vi "Get Pi Data.vi"() -> ()   [LabVIEW 2020]
panel:
  out "standard error":string
  out "standard output":string="Active Internet connections (w/o servers)\nProto Recv-Q Send-Q Local Address           Foreign Address         State       \ntcp        0      0 localhost:39876         localhost:41539         ESTABLISHED \ntcp        0    232 192.168.1.102:3079      192.168.1.101:62664     ESTABLISHED \ntcp        0      0 localhost:41539         localhost:39876         ESTABLISHED \nActive UNIX domain sockets (w/o servers)\nProto RefCnt Flags       Type       State         I-Node Path\nunix  2      [ ]         DGRAM                     19720 /run/user/1000/systemd/notify\nunix  4      [ ]         DGRAM                     17418 /var/run/wpa_supplicant/wlan0\nunix  2      [ ]         DGRAM                     17427 /var/run/wpa_supplicant/p2p-dev-wlan0\nunix  2      [ ]         DGRAM                     15198 /tmp/.vncserver-license/0.504\nunix  3      [ ]         DGRAM                      5458 /run/systemd/notify\nunix  2      [ ]         DGRAM                     19551 /run/user/0/systemd/notify\nunix  8      [ ]         DGRAM                      5481 /run/systemd/journal/socket\nunix  20     [ ]         DGRAM                      5493 /run/systemd/journal/dev-log\nunix  2      [ ]         DGRAM                      5517 /run/systemd/journal/syslog\nunix  2      [ ]         DGRAM                     23574 /tmp/dhcpcd-pi/libdhcpcd-wpa-888.0\nunix  2      [ ]         DGRAM                     23575 /tmp/dhcpcd-pi/libdhcpcd-wpa-888.1\nunix  3      [ ]         STREAM     CONNECTED      20302 \nunix  3      [ ]         STREAM     CONNECTED      18013 \nunix  3      [ ]         STREAM     CONNECTED      17093 \nunix  3      [ ]         STREAM     CONNECTED      13957 \nunix  3      [ ]         STREAM     CONNECTED      21078 @/tmp/.X11-unix/X0\nunix  3      [ ]         STREAM     CONNECTED      22652 \nunix  3      [ ]         STREAM     CONNECTED      21440 /run/user/1000/bus\nunix  3      [ ]         STREAM     CONNECTED      20321 @/tmp/.X11-unix/X0\nunix  3      [ ]         STREAM     CONNECTED      19605 /var/run/dbus/system_bus_socket\nunix  3      [ ]         STREAM     CONNECTED      17472 \nunix  2      [ ]         DGRAM                     17271 \nunix  3      [ ]         STREAM     CONNECTED      20299 \nunix  3      [ ]         STREAM     CONNECTED      17782 /run/systemd/journal/stdout\nunix  3      [ ]         STREAM     CONNECTED      14033 \nunix  3      [ ]         STREAM     CONNECTED      17473 /var/run/dbus/system_bus_socket\nunix  3      [ ]         STREAM     CONNECTED      18014 \nunix  3      [ ]         STREAM     CONNECTED      13772 \nunix  3      [ ]         STREAM     CONNECTED      21437 /run/user/1000/bus\nunix  2      [ ]         DGRAM                     17486 \nunix  3      [ ]         STREAM     CONNECTED      20350 /var/run/dbus/system_bus_socket\nunix  2      [ ]         DGRAM                     18729 \nunix  3      [ ]         STREAM     CONNECTED      18114 \nunix  2      [ ]         DGRAM                     17761 \nunix  3      [ ]         STREAM     CONNECTED      13705 \nunix  3      [ ]         STREAM     CONNECTED      18188 /run/systemd/journal/stdout\nunix  2      [ ]         DGRAM                     18697 \nunix  3      [ ]         STREAM     CONNECTED      17270 \nunix  2      [ ]         DGRAM                     13792 \nunix  3      [ ]         STREAM     CONNECTED      21410 \nunix  3      [ ]         STREAM     CONNECTED      18397 /run/user/1000/bus\nunix  3      [ ]         STREAM     CONNECTED      20344 /var/run/dbus/system_bus_socket\nunix  3      [ ]         STREAM     CONNECTED      21127 \nunix  3      [ ]         STREAM     CONNECTED      17009 \nunix  3      [ ]         STREAM     CONNECTED      22631 \nunix  3      [ ]         STREAM     CONNECTED      20264 \nunix  3      [ ]         STREAM     CONNECTED      19600 @/tmp/.X11-unix/X0\nunix  3      [ ]         STREAM     CONNECTED      16668 \nunix  3      [ ]         STREAM     CONNECTED      18410 /run/user/1000/bus\nunix  3      [ ]         STREAM     CONNECTED      18689 \nunix  3      [ ]         STREAM     CONNECTED      18696 \nunix  3      [ ]         STREAM     CONNECTED      17276 \nunix  3      [ ]         STREAM     CONNECTED      17010 /run/systemd/journal/stdout\nunix  3      [ ]         STREAM     CONNECTED      14034 /run/systemd/journal/stdout\nunix  3      [ ]         STREAM     CONNECTED      21326 /run/user/1000/bus\nunix  3      [ ]         STREAM     CONNECTED      22653 \nunix  3      [ ]         STREAM     CONNECTED      22630 \nunix  3      [ ]         STREAM     CONNECTED      16636 \nunix  3      [ ]         STREAM     CONNECTED      14907 \nunix  3      [ ]         STREAM     CONNECTED      14912 /var/run/dbus/system_bus_socket\nunix  3      [ ]         STREAM     CONNECTED      17277 /var/run/dbus/system_bus_socket\nunix  2      [ ]         DGRAM                     16633 \nunix  3      [ ]         STREAM     CONNECTED      18395 /run/systemd/journal/stdout\nunix  3      [ ]         STREAM     CONNECTED      15137 \nunix  3      [ ]         STREAM     CONNECTED      20314 \nunix  3      [ ]         STREAM     CONNECTED      14906 \nunix  3      [ ]         STREAM     CONNECTED      14911 /var/run/dbus/system_bus_socket\nunix  3      [ ]         STREAM     CONNECTED      17094 /run/systemd/journal/stdout\nunix  3      [ ]         STREAM     CONNECTED      14142 \nunix  3      [ ]         STREAM     CONNECTED      21596 /run/user/1000/bus\nunix  3      [ ]         STREAM     CONNECTED      18501 \nunix  2      [ ]         DGRAM                     14137 \nunix  3      [ ]         STREAM     CONNECTED      21604 @/dbus-vfs-daemon/socket-T8U37b0E\nunix  3      [ ]         STREAM     CONNECTED      18128 \nunix  3      [ ]         STREAM     CONNECTED      17437 /run/systemd/journal/stdout\nunix  3      [ ]         STREAM     CONNECTED      21304 /run/user/1000/bus\nunix  3      [ ]         STREAM     CONNECTED      16635 \nunix  3      [ ]         STREAM     CONNECTED      14909 /var/run/dbus/system_bus_socket\nunix  3      [ ]         STREAM     CONNECTED      18910 \nunix  3      [ ]         STREAM     CONNECTED      13774 /run/systemd/journal/stdout\nunix  3      [ ]         STREAM     CONNECTED      18899 \nunix  3      [ ]         STREAM     CONNECTED      17450 /var/run/dbus/system_bus_socket\nunix  2      [ ]         DGRAM                     16602 \nunix  3      [ ]         STREAM     CONNECTED      20311 \nunix  3      [ ]         STREAM     CONNECTED      18909 \nunix  3      [ ]         STREAM     CONNECTED      14118 /run/systemd/journal/stdout\nunix  3      [ ]         STREAM     CONNECTED      19260 /run/user/1000/bus\nunix  3      [ ]         STREAM     CONNECTED      19597 @/tmp/.X11-unix/X0\nunix  2      [ ]         DGRAM                     14041 \nunix  3      [ ]         STREAM     CONNECTED      15099 \nunix  3      [ ]         STREAM     CONNECTED      18212 /run/systemd/journal/stdout\nunix  3      [ ]         STREAM     CONNECTED      14117 \nunix  3      [ ]         STREAM     CONNECTED      21444 /run/user/1000/bus\nunix  3      [ ]         STREAM     CONNECTED      15115 \nunix  3      [ ]         STREAM     CONNECTED      14962 /run/systemd/journal/stdout\nunix  3      [ ]         STREAM     CONNECTED      13958 /run/systemd/journal/stdout\nunix  2      [ ]         DGRAM                     18007 \nunix  3      [ ]         STREAM     CONNECTED      20309 \nunix  3      [ ]         STREAM     CONNECTED      21527 \nunix  3      [ ]         STREAM     CONNECTED      17477 /var/run/dbus/system_bus_socket\nunix  3      [ ]         STREAM     CONNECTED      19558 /var/run/dbus/system_bus_socket\nunix  3      [ ]         STREAM     CONNECTED      15158 \nunix  2      [ ]         DGRAM                      7126 \nunix  2      [ ]         DGRAM                     19704 \nunix  3      [ ]         STREAM     CONNECTED      21272 \nunix  3      [ ]         STREAM     CONNECTED      14781 \nunix  2      [ ]         STREAM     CONNECTED      15142 \nunix  3      [ ]         DGRAM                     19554 \nunix  3      [ ]         STREAM     CONNECTED      14615 \nunix  3      [ ]         STREAM     CONNECTED      16076 \nunix  3      [ ]         DGRAM                     19553 \nunix  3      [ ]         STREAM     CONNECTED      19455 \nunix  3      [ ]         STREAM     CONNECTED      14927 /run/systemd/journal/stdout\nunix  3      [ ]         STREAM     CONNECTED      22628 \nunix  2      [ ]         STREAM     CONNECTED      15150 \nunix  3      [ ]         STREAM     CONNECTED      19557 \nunix  3      [ ]         STREAM     CONNECTED      13595 /run/systemd/journal/stdout\nunix  3      [ ]         STREAM     CONNECTED      14913 /var/run/dbus/system_bus_socket\nunix  3      [ ]         STREAM     CONNECTED      13813 /run/systemd/journal/stdout\nunix  3      [ ]         STREAM     CONNECTED      19726 \nunix  3      [ ]         STREAM     CONNECTED      21267 @/tmp/.X11-unix/X0\nunix  2      [ ]         DGRAM                     15196 \nunix  3      [ ]         STREAM     CONNECTED      16216 /var/run/dbus/system_bus_socket\nunix  2      [ ]         DGRAM                     14689 \nunix  3      [ ]         STREAM     CONNECTED      19454 \nunix  3      [ ]         STREAM     CONNECTED      21275 @/tmp/.X11-unix/X0\nunix  2      [ ]         STREAM     CONNECTED      15206 \nunix  2      [ ]         DGRAM                     19701 \nunix  3      [ ]         STREAM     CONNECTED      17279 \nunix  3      [ ]         STREAM     CONNECTED      17481 /var/run/dbus/system_bus_socket\nunix  3      [ ]         STREAM     CONNECTED      20948 /run/systemd/journal/stdout\nunix  3      [ ]         STREAM     CONNECTED      15160 \nunix  3      [ ]         STREAM     CONNECTED      19695 \nunix  3      [ ]         STREAM     CONNECTED      18331 \nunix  3      [ ]         STREAM     CONNECTED      17390 /var/run/dbus/system_bus_socket\nunix  3      [ ]         STREAM     CONNECTED      10394 /run/systemd/journal/stdout\nunix  3      [ ]         STREAM     CONNECTED      21599 /run/user/1000/bus\nunix  3      [ ]         STREAM     CONNECTED      16381 \nunix  3      [ ]         STREAM     CONNECTED       8029 \nunix  3      [ ]         STREAM     CONNECTED      21269 \nunix  3      [ ]         STREAM     CONNECTED      18348 \nunix  3      [ ]         STREAM     CONNECTED      22697 /var/run/dhcpcd.unpriv.sock\nunix  3      [ ]         DGRAM                     21355 \nunix  3      [ ]         STREAM     CONNECTED      22696 /var/run/dhcpcd.unpriv.sock\nunix  3      [ ]         STREAM     CONNECTED      21601 /run/user/1000/bus\nunix  3      [ ]         STREAM     CONNECTED      16323 \nunix  3      [ ]         STREAM     CONNECTED      23571 \nunix  3      [ ]         STREAM     CONNECTED      14910 /var/run/dbus/system_bus_socket\nunix  3      [ ]         STREAM     CONNECTED      23570 \nunix  3      [ ]         STREAM     CONNECTED      18288 \nunix  3      [ ]         STREAM     CONNECTED      16235 \nunix  3      [ ]         STREAM     CONNECTED      15851 \nunix  3      [ ]         STREAM     CONNECTED      21438 /run/systemd/journal/stdout\nunix  3      [ ]         STREAM     CONNECTED      17470 /var/run/dbus/system_bus_socket\nunix  3      [ ]         STREAM     CONNECTED      18415 \nunix  2      [ ]         DGRAM                     20124 \nunix  3      [ ]         STREAM     CONNECTED      18359 \nunix  3      [ ]         STREAM     CONNECTED      16236 \nunix  3      [ ]         STREAM     CONNECTED      18329 \nunix  3      [ ]         DGRAM                      8037 \nunix  3      [ ]         STREAM     CONNECTED      16382 \nunix  2      [ ]         DGRAM                      8033 \nunix  3      [ ]         STREAM     CONNECTED      21446 /run/systemd/journal/stdout\nunix  3      [ ]         STREAM     CONNECTED      17466 /var/run/dbus/system_bus_socket\nunix  3      [ ]         DGRAM                      8036 \nunix  3      [ ]         STREAM     CONNECTED      16504 \nunix  2      [ ]         DGRAM                     15838 \nunix  3      [ ]         STREAM     CONNECTED      18202 \nunix  3      [ ]         STREAM     CONNECTED      21270 @/tmp/.X11-unix/X0\nunix  3      [ ]         STREAM     CONNECTED      21372 @/tmp/.X11-unix/X0\nunix  3      [ ]         STREAM     CONNECTED      20119 /var/run/dbus/system_bus_socket\nunix  3      [ ]         STREAM     CONNECTED      21426 /run/systemd/journal/stdout\nunix  3      [ ]         STREAM     CONNECTED      16577 \nunix  3      [ ]         STREAM     CONNECTED      18252 \nunix  2      [ ]         DGRAM                     19261 \nunix  3      [ ]         STREAM     CONNECTED      21351 \nunix  3      [ ]         STREAM     CONNECTED      21428 /run/user/1000/bus\nunix  3      [ ]         STREAM     CONNECTED      17464 /var/run/dbus/system_bus_socket\nunix  3      [ ]         STREAM     CONNECTED      14037 /run/systemd/journal/stdout\nunix  3      [ ]         STREAM     CONNECTED      18179 \nunix  3      [ ]         STREAM     CONNECTED      18414 \nunix  3      [ ]         STREAM     CONNECTED      18360 /var/run/dbus/system_bus_socket\nunix  3      [ ]         DGRAM                     21356 \nunix  3      [ ]         STREAM     CONNECTED      18180 /run/systemd/journal/stdout\nunix  3      [ ]         STREAM     CONNECTED      20165 @/tmp/.X11-unix/X0\nunix  3      [ ]         STREAM     CONNECTED      20160 @/tmp/.X11-unix/X0\nunix  3      [ ]         STREAM     CONNECTED      18364 \nunix  3      [ ]         STREAM     CONNECTED      13964 /run/systemd/journal/stdout\nunix  3      [ ]         STREAM     CONNECTED      18250 \nunix  3      [ ]         STREAM     CONNECTED      21531 \nunix  3      [ ]         STREAM     CONNECTED      21160 \nunix  3      [ ]         STREAM     CONNECTED      18912 /run/user/1000/bus\nunix  3      [ ]         STREAM     CONNECTED      20882 \nunix  3      [ ]         STREAM     CONNECTED      18022 /run/systemd/journal/stdout\nunix  3      [ ]         DGRAM                     15593 \nunix  3      [ ]         STREAM     CONNECTED      21541 \nunix  3      [ ]         STREAM     CONNECTED      21648 \nunix  3      [ ]         DGRAM                     15592 \nunix  3      [ ]         STREAM     CONNECTED      20116 \nunix  3      [ ]         DGRAM                     19722 \nunix  3      [ ]         DGRAM                     15591 \nunix  3      [ ]         STREAM     CONNECTED      21540 \nunix  3      [ ]         STREAM     CONNECTED      14908 /var/run/dbus/system_bus_socket\nunix  3      [ ]         STREAM     CONNECTED      13506 /run/systemd/journal/stdout\nunix  3      [ ]         STREAM     CONNECTED      21679 \nunix  3      [ ]         STREAM     CONNECTED      18646 /run/systemd/journal/stdout\nunix  3      [ ]         STREAM     CONNECTED      19268 /run/user/1000/bus\nunix  2      [ ]         DGRAM                     15976 \nunix  3      [ ]         STREAM     CONNECTED      20115 \nunix  2      [ ]         DGRAM                     20891 \nunix  3      [ ]         STREAM     CONNECTED      20092 \nunix  3      [ ]         STREAM     CONNECTED      15689 \nunix  3      [ ]         STREAM     CONNECTED      13564 /run/systemd/journal/stdout\nunix  3      [ ]         STREAM     CONNECTED      13073 \nunix  2      [ ]         DGRAM                     20894 \nunix  3      [ ]         STREAM     CONNECTED      18429 /run/user/1000/menu-cached-:0\nunix  3      [ ]         STREAM     CONNECTED      20118 \nunix  3      [ ]         STREAM     CONNECTED      19765 \nunix  3      [ ]         STREAM     CONNECTED      15622 \nunix  3      [ ]         DGRAM                     19723 \nunix  3      [ ]         STREAM     CONNECTED      21420 /run/user/1000/bus\nunix  3      [ ]         STREAM     CONNECTED      21229 /run/user/1000/bus\nunix  3      [ ]         STREAM     CONNECTED      21044 /var/run/dbus/system_bus_socket\nunix  3      [ ]         STREAM     CONNECTED      17775 /var/run/dbus/system_bus_socket\nunix  3      [ ]         STREAM     CONNECTED      21551 \nunix  3      [ ]         STREAM     CONNECTED      19973 \nunix  3      [ ]         STREAM     CONNECTED      18401 /run/user/1000/pulse/native\nunix  3      [ ]         STREAM     CONNECTED      21412 \nunix  3      [ ]         STREAM     CONNECTED      21442 /run/systemd/journal/stdout\nunix  3      [ ]         STREAM     CONNECTED      19967 \nunix  3      [ ]         STREAM     CONNECTED      15979 \nunix  3      [ ]         STREAM     CONNECTED      21590 \nunix  3      [ ]         STREAM     CONNECTED      21021 /run/systemd/journal/stdout\nunix  2      [ ]         DGRAM                     15831 \nunix  3      [ ]         DGRAM                      5460 \nunix  3      [ ]         STREAM     CONNECTED      19392 /run/user/1000/bus\nunix  3      [ ]         STREAM     CONNECTED      21161 @/tmp/.X11-unix/X0\nunix  2      [ ]         DGRAM                     19971 \nunix  3      [ ]         DGRAM                     15590 \nunix  3      [ ]         STREAM     CONNECTED      21227 @/tmp/.X11-unix/X0\nunix  2      [ ]         DGRAM                      5548 \nunix  3      [ ]         STREAM     CONNECTED      21413 /var/run/dbus/system_bus_socket\nunix  2      [ ]         DGRAM                     15588 \nunix  3      [ ]         DGRAM                      5461 \nunix  3      [ ]         STREAM     CONNECTED      20108 \n\u001b[H\u001b[JMem: 447224K used, 499812K free, 13980K shrd, 43740K buff, 221764K cached\nCPU:   0% usr   2% sys   0% nic  97% idle   0% io   0% irq   0% sirq\nLoad average: 0.02 0.04 0.09 1/236 2623\n\u001b[7m  PID  PPID USER     STAT   VSZ %VSZ %CPU COMMAND\u001b[m\n 2623  2621 root     R     2796   0%   2% top -n 1\n  972   747 pi       S<    442m  48%   0% /usr/bin/pulseaudio --daemonize=no\n  888   775 pi       S     412m  45%   0% lxpanel --profile LXDE-pi\n  565   499 root     S     268m  29%   0% /usr/lib/xorg/Xorg :0 -seat seat0 -aut\n  889   775 pi       S     136m  15%   0% pcmanfm --desktop --profile LXDE-pi\n  991   747 pi       S    97900  10%   0% /usr/lib/gvfs/gvfs-udisks2-volume-moni\n  438     1 root     S    65356   7%   0% /usr/lib/udisks2/udisksd\n  882   775 pi       S    62296   7%   0% openbox --config-file /home/pi/.config\n  868   747 pi       S    56756   6%   0% /usr/lib/gvfs/gvfsd-fuse /run/user/100\n  775   736 pi       S    56212   6%   0% /usr/bin/lxsession -s LXDE-pi -e LXDE\n  995   747 pi       S    56028   6%   0% /usr/lib/gvfs/gvfs-afc-volume-monitor\n 1020   850 pi       S    55112   6%   0% /usr/lib/gvfs/gvfsd-trash --spawner :1\n  886   775 pi       S    47136   5%   0% lxpolkit\n  909     1 pi       S    46324   5%   0% {applet.py} /usr/bin/python3 /usr/shar\n  850   747 pi       S    43412   5%   0% /usr/lib/gvfs/gvfsd\n 1004   747 pi       S    41696   4%   0% /usr/lib/gvfs/gvfs-gphoto2-volume-moni\n  500     1 root     S    41536   4%   0% /usr/lib/policykit-1/polkitd --no-debu\n  494     1 root     S    40492   4%   0% /usr/sbin/cups-browsed\n 1000   747 pi       S    40128   4%   0% /usr/lib/gvfs/gvfs-mtp-volume-monitor\n 1013   747 pi       S    40104   4%   0% /usr/lib/gvfs/gvfs-goa-volume-monitor\r\n  PID USER       VSZ STAT COMMAND\n    1 root     33820 S    {systemd} /sbin/init splash\n    2 root         0 SW   [kthreadd]\n    3 root         0 IW<  [rcu_gp]\n    4 root         0 IW<  [rcu_par_gp]\n    8 root         0 IW<  [mm_percpu_wq]\n    9 root         0 SW   [ksoftirqd/0]\n   10 root         0 IW   [rcu_sched]\n   11 root         0 SW   [migration/0]\n   12 root         0 SW   [cpuhp/0]\n   13 root         0 SW   [cpuhp/1]\n   14 root         0 SW   [migration/1]\n   15 root         0 SW   [ksoftirqd/1]\n   18 root         0 SW   [cpuhp/2]\n   19 root         0 SW   [migration/2]\n   20 root         0 SW   [ksoftirqd/2]\n   23 root         0 SW   [cpuhp/3]\n   24 root         0 SW   [migration/3]\n   25 root         0 SW   [ksoftirqd/3]\n   28 root         0 SW   [kdevtmpfs]\n   29 root         0 IW<  [netns]\n   32 root         0 SW   [kauditd]\n   33 root         0 SW   [khungtaskd]\n   34 root         0 SW   [oom_reaper]\n   35 root         0 IW<  [writeback]\n   36 root         0 SW   [kcompactd0]\n   54 root         0 IW<  [kblockd]\n   55 root         0 IW<  [blkcg_punt_bio]\n   56 root         0 SW   [watchdogd]\n   59 root         0 IW<  [rpciod]\n   60 root         0 IW<  [kworker/u9:0-hc]\n   61 root         0 IW<  [xprtiod]\n   62 root         0 SW   [kswapd0]\n   63 root         0 IW<  [nfsiod]\n   64 root         0 IW<  [iscsi_eh]\n   65 root         0 IW<  [dwc_otg]\n   66 root         0 IW<  [DWC Notificatio]\n   68 root         0 SW<  [vchiq-slot/0]\n   69 root         0 SW<  [vchiq-recy/0]\n   70 root         0 SW<  [vchiq-sync/0]\n   71 root         0 SW   [vchiq-keep/0]\n   72 root         0 SW<  [SMIO]\n   73 root         0 IW   [kworker/2:2-mm_]\n   75 root         0 IW<  [mmc_complete]\n   76 root         0 IW<  [kworker/2:1H-kb]\n   77 root         0 IW<  [kworker/0:1H-mm]\n   78 root         0 IW<  [kworker/1:1H-kb]\n   80 root         0 SW   [jbd2/mmcblk0p2-]\n   81 root         0 IW<  [ext4-rsv-conver]\n   82 root         0 IW<  [ipv6_addrconf]\n   83 root         0 IW   [kworker/0:2-eve]\n   86 root         0 IW   [kworker/1:3-eve]\n   89 root         0 IW<  [kworker/3:1H-kb]\n  102 root         0 SW   [scsi_eh_0]\n  103 root         0 IW<  [scsi_tmf_0]\n  104 root         0 SW   [usb-storage]\n  110 root         0 IW<  [kworker/2:2H-kb]\n  115 root         0 IW<  [kworker/1:2H-kb]\n  116 root     19140 S    /lib/systemd/systemd-journald\n  132 root         0 SW   [irq/166-usb-001]\n  140 root         0 IW   [kworker/3:3-eve]\n  151 root     18564 S    /lib/systemd/systemd-udevd\n  173 root         0 SW<  [SMIO]\n  176 root         0 SW   [spi0]\n  187 root         0 IW<  [mmal-vchiq]\n  189 root         0 IW<  [mmal-vchiq]\n  191 root         0 IW<  [mmal-vchiq]\n  193 root         0 IW<  [mmal-vchiq]\n  219 root         0 IW<  [uas]\n  229 root         0 IW<  [cfg80211]\n  233 root         0 IW<  [brcmf_wq/mmc1:0]\n  234 root         0 SW   [brcmf_wdog/mmc1]\n  339 systemd- 22412 S    /lib/systemd/systemd-timesyncd\n  379 root     13156 S    /lib/systemd/systemd-logind\n  397 root     25512 S    /usr/sbin/rsyslogd -n -iNONE\n  398 root     11768 SN   /usr/sbin/alsactl -E HOME=/run/alsa -s -n 19 -c rdae\n  405 root     27656 S    /usr/sbin/rngd -r /dev/hwrng\n  413 messageb  6972 S    /usr/bin/dbus-daemon --system --address=systemd: --n\n  430 root     10740 S    /sbin/wpa_supplicant -u -s -O /run/wpa_supplicant\n  438 root     65356 S    /usr/lib/udisks2/udisksd\n  441 root      7976 S    /usr/sbin/cron -f\n  442 nobody    4320 S    /usr/sbin/thd --triggers /etc/triggerhappy/triggers.\n  444 root     27640 S    /usr/sbin/cupsd -l\n  448 avahi     5904 S    avahi-daemon: running [raspberrypi.local]\n  462 avahi     5772 S    avahi-daemon: chroot helper\n  463 root      2904 S    /sbin/dhcpcd -q -b\n  486 root     34376 S    {NISysServer.py} /usr/bin/python /usr/sbin/NISysServ\n  493 root      8628 S    /usr/bin/vncserver-x11-serviced -fg\n  494 root     40492 S    /usr/sbin/cups-browsed\n  499 root     40100 S    /usr/sbin/lightdm\n  500 root     41536 S    /usr/lib/policykit-1/polkitd --no-debug\n  504 root     32728 S    /usr/bin/vncserver-x11-core -service\n  513 root     11132 S    wpa_supplicant -B -c/etc/wpa_supplicant/wpa_supplica\n  524 root     10724 S    /usr/sbin/sshd -D\n  528 lp       13832 S    /usr/lib/cups/notifier/dbus dbus://\n  530 lp       13832 S    /usr/lib/cups/notifier/dbus dbus://\n  531 lp       13832 S    /usr/lib/cups/notifier/dbus dbus://\n  532 lp       13832 S    /usr/lib/cups/notifier/dbus dbus://\n  565 root      268m S    /usr/lib/xorg/Xorg :0 -seat seat0 -auth /var/run/lig\n  566 root      6616 S    /sbin/agetty -o -p -- \\u --keep-baud 115200,38400,96\n  567 root      5620 S    /bin/login -f\n  614 root     11480 S    /usr/bin/vncagent service 15\n  703 root     14700 S    /lib/systemd/systemd --user\n  704 root     16920 S    (sd-pam)\n  717 root     38860 S    {MainAppThread} ./lvrt\n  736 root     32400 S    lightdm --session-child 14 17\n  747 pi       14808 S    /lib/systemd/systemd --user\n  749 pi       16920 S    (sd-pam)\n  775 pi       56212 S    /usr/bin/lxsession -s LXDE-pi -e LXDE\n  783 pi        6544 S    /usr/bin/dbus-daemon --session --address=systemd: --\n  796 root      2140 S    /usr/bin/hciattach /dev/serial1 bcm43xx 3000000 flow\n  798 root         0 IW<  [kworker/u9:2-hc]\n  820 root      9536 S    /usr/lib/bluetooth/bluetoothd\n  822 pi        4520 S    /usr/bin/ssh-agent x-session-manager\n  846 pi        8492 S    -bash\n  850 pi       43412 S    /usr/lib/gvfs/gvfsd\n  868 pi       56756 S    /usr/lib/gvfs/gvfsd-fuse /run/user/1000/gvfs -f -o b\n  882 pi       62296 S    openbox --config-file /home/pi/.config/openbox/lxde-\n  886 pi       47136 S    lxpolkit\n  888 pi        412m S    lxpanel --profile LXDE-pi\n  889 pi        136m S    pcmanfm --desktop --profile LXDE-pi\n  895 pi        4520 S    /usr/bin/ssh-agent -s\n  909 pi       46324 S    {applet.py} /usr/bin/python3 /usr/share/system-confi\n  942 pi       32024 S    /usr/bin/vncserverui service 16\n  972 pi        442m S<   /usr/bin/pulseaudio --daemonize=no\n  986 rtkit    23188 SN   /usr/lib/rtkit/rtkit-daemon\n  989 pi       31740 S    /usr/bin/vncserverui -statusicon 5\n  991 pi       97900 S    /usr/lib/gvfs/gvfs-udisks2-volume-monitor\n  995 pi       56028 S    /usr/lib/gvfs/gvfs-afc-volume-monitor\n 1000 pi       40128 S    /usr/lib/gvfs/gvfs-mtp-volume-monitor\n 1004 pi       41696 S    /usr/lib/gvfs/gvfs-gphoto2-volume-monitor\n 1008 pi       28696 S    /usr/lib/menu-cache/menu-cached /run/user/1000/menu-\n 1013 pi       40104 S    /usr/lib/gvfs/gvfs-goa-volume-monitor\n 1020 pi       55112 S    /usr/lib/gvfs/gvfsd-trash --spawner :1.4 /org/gtk/gv\n 1030 root         0 SW<  [krfcommd]\n 1054 pi       30980 S    /usr/lib/gvfs/gvfsd-metadata\n 1517 root         0 IW   [kworker/u8:0-cf]\n 1522 root         0 IW<  [kworker/0:0H]\n 1655 root         0 IW<  [kworker/3:0H]\n 2367 root         0 IW   [kworker/u8:1-fl]\n 2494 root         0 IW   [kworker/2:0-eve]\n 2507 root         0 IW   [kworker/0:0-eve]\n 2511 root         0 IW   [kworker/1:0-eve]\n 2512 root         0 IW   [kworker/3:1-mm_]\n 2530 root         0 IW   [kworker/u8:2-br]\n 2578 root         0 IW   [kworker/2:1-eve]\n 2579 root         0 IW<  [kworker/2:0H]\n 2598 root         0 IW   [kworker/0:1-mm_]\n 2619 root         0 IW   [kworker/2:3-mm_]\n 2620 root         0 IW<  [kworker/1:0H]\n 2621 root      3060 S    /bin/sh -c netstat top -n 1 ps hostname cat /proc/me\n 2624 root      2888 R    ps\nraspberrypi\nMemTotal:         947036 kB\nMemFree:          499756 kB\nMemAvailable:     701388 kB\nBuffers:           43740 kB\nCached:           221764 kB\nSwapCached:            0 kB\nActive:           210792 kB\nInactive:         149504 kB\nActive(anon):     108932 kB\nInactive(anon):    13600 kB\nActive(file):     101860 kB\nInactive(file):   135904 kB\nUnevictable:       31916 kB\nMlocked:           31916 kB\nSwapTotal:        102396 kB\nSwapFree:         102396 kB\nDirty:                 0 kB\nWriteback:             0 kB\nAnonPages:        126872 kB\nMapped:           110976 kB\nShmem:             13980 kB\nKReclaimable:      17848 kB\nSlab:              34668 kB\nSReclaimable:      17848 kB\nSUnreclaim:        16820 kB\nKernelStack:        1928 kB\nPageTables:         4260 kB\nNFS_Unstable:          0 kB\nBounce:                0 kB\nWritebackTmp:          0 kB\nCommitLimit:      575912 kB\nCommitted_AS:     979260 kB\nVmallocTotal:    1114112 kB\nVmallocUsed:        3672 kB\nVmallocChunk:          0 kB\nPercpu:              464 kB\nCmaTotal:          65536 kB\nCmaFree:           63124 kB\nmajor minor  #blocks  name\n\n   1        0       4096 ram0\n   1        1       4096 ram1\n   1        2       4096 ram2\n   1        3       4096 ram3\n   1        4       4096 ram4\n   1        5       4096 ram5\n   1        6       4096 ram6\n   1        7       4096 ram7\n   1        8       4096 ram8\n   1        9       4096 ram9\n   1       10       4096 ram10\n   1       11       4096 ram11\n   1       12       4096 ram12\n   1       13       4096 ram13\n   1       14       4096 ram14\n   1       15       4096 ram15\n 179        0   30707712 mmcblk0\n 179        1     262144 mmcblk0p1\n 179        2   30441472 mmcblk0p2\n   8        0   31328320 sda\n   8        1   31328208 sda1\nFilesystem                Size      Used Available Use% Mounted on\n/dev/root                28.5G      3.0G     24.3G  11% /\ndevtmpfs                429.9M         0    429.9M   0% /dev\n/dev/root                28.5G      3.0G     24.3G  11% /home\n/dev/root                28.5G      3.0G     24.3G  11% /tmp\n/dev/mmcblk0p1          252.0M     61.8M    190.2M  25% /boot\n/dev/root                28.5G      3.0G     24.3G  11% /media\n/dev/root                28.5G      3.0G     24.3G  11% /mnt\ntmpfs                   462.4M      6.3M    456.1M   1% /run\ntmpfs                     5.0M      4.0K      5.0M   0% /run/lock\n/dev/root                28.5G      3.0G     24.3G  11% /lib/firmware\nLinux version 5.4.79-v7+ (dom@buildbot) (gcc version 8.4.0 (Ubuntu/Linaro 8.4.0-3ubuntu1)) #1373 SMP Mon Nov 23 13:22:33 GMT 2020\nLinux raspberrypi 5.4.79-v7+ #1373 SMP Mon Nov 23 13:22:33 GMT 2020 armv7l GNU/Linux\nDisk /dev/mmcblk0: 29 GB, 31444697088 bytes, 61415424 sectors\n959616 cylinders, 4 heads, 16 sectors/track\nUnits: sectors of 1 * 512 = 512 bytes\n\nDevice       Boot StartCHS    EndCHS        StartLBA     EndLBA    Sectors  Size Id Type\n/dev/mmcblk0p1    64,0,1      1023,3,32         8192     532479     524288  256M  c Win95 FAT32 (LBA)\n/dev/mmcblk0p2    1023,3,32   1023,63,32      532480   61415423   60882944 29.0G 83 Linux\nDisk /dev/sda: 30 GB, 32080200192 bytes, 62656641 sectors\n3900 cylinders, 255 heads, 63 sectors/track\nUnits: sectors of 1 * 512 = 512 bytes\n\nDevice  Boot StartCHS    EndCHS        StartLBA     EndLBA    Sectors  Size Id Type\n/dev/sda1    0,3,36      1023,254,63        224   62656640   62656417 29.8G  7 HPFS/NTFS\neth0      Link encap:Ethernet  HWaddr B8:27:EB:17:35:B9  \n          inet addr:192.168.1.102  Bcast:192.168.1.255  Mask:255.255.255.0\n          inet6 addr: fe80::16f4:3014:dae5:8846/64 Scope:Link\n          UP BROADCAST RUNNING MULTICAST  MTU:1500  Metric:1\n          RX packets:320699 errors:0 dropped:0 overruns:0 frame:0\n          TX packets:13886 errors:0 dropped:0 overruns:0 carrier:0\n          collisions:0 txqueuelen:1000 \n          RX bytes:401388444 (382.7 MiB)  TX bytes:2385408 (2.2 MiB)\n\nlo        Link encap:Local Loopback  \n          inet addr:127.0.0.1  Mask:255.0.0.0\n          inet6 addr: ::1/128 Scope:Host\n          UP LOOPBACK RUNNING  MTU:65536  Metric:1\n          RX packets:35 errors:0 dropped:0 overruns:0 frame:0\n          TX packets:35 errors:0 dropped:0 overruns:0 carrier:0\n          collisions:0 txqueuelen:1000 \n          RX bytes:2576 (2.5 KiB)  TX bytes:2576 (2.5 KiB)\n\nwlan0     Link encap:Ethernet  HWaddr B8:27:EB:42:60:EC  \n          UP BROADCAST MULTICAST  MTU:1500  Metric:1\n          RX packets:0 errors:0 dropped:0 overruns:0 frame:0\n          TX packets:0 errors:0 dropped:0 overruns:0 carrier:0\n          collisions:0 txqueuelen:1000 \n          RX bytes:0 (0.0 B)  TX bytes:0 (0.0 B)\n\n"
  in  "command line":string="netstat\ntop -n 1\nps\nhostname\ncat /proc/meminfo\ncat /proc/partitions\ndf -h\ncat /proc/version\nuname -a\nfdisk -l\nifconfig"
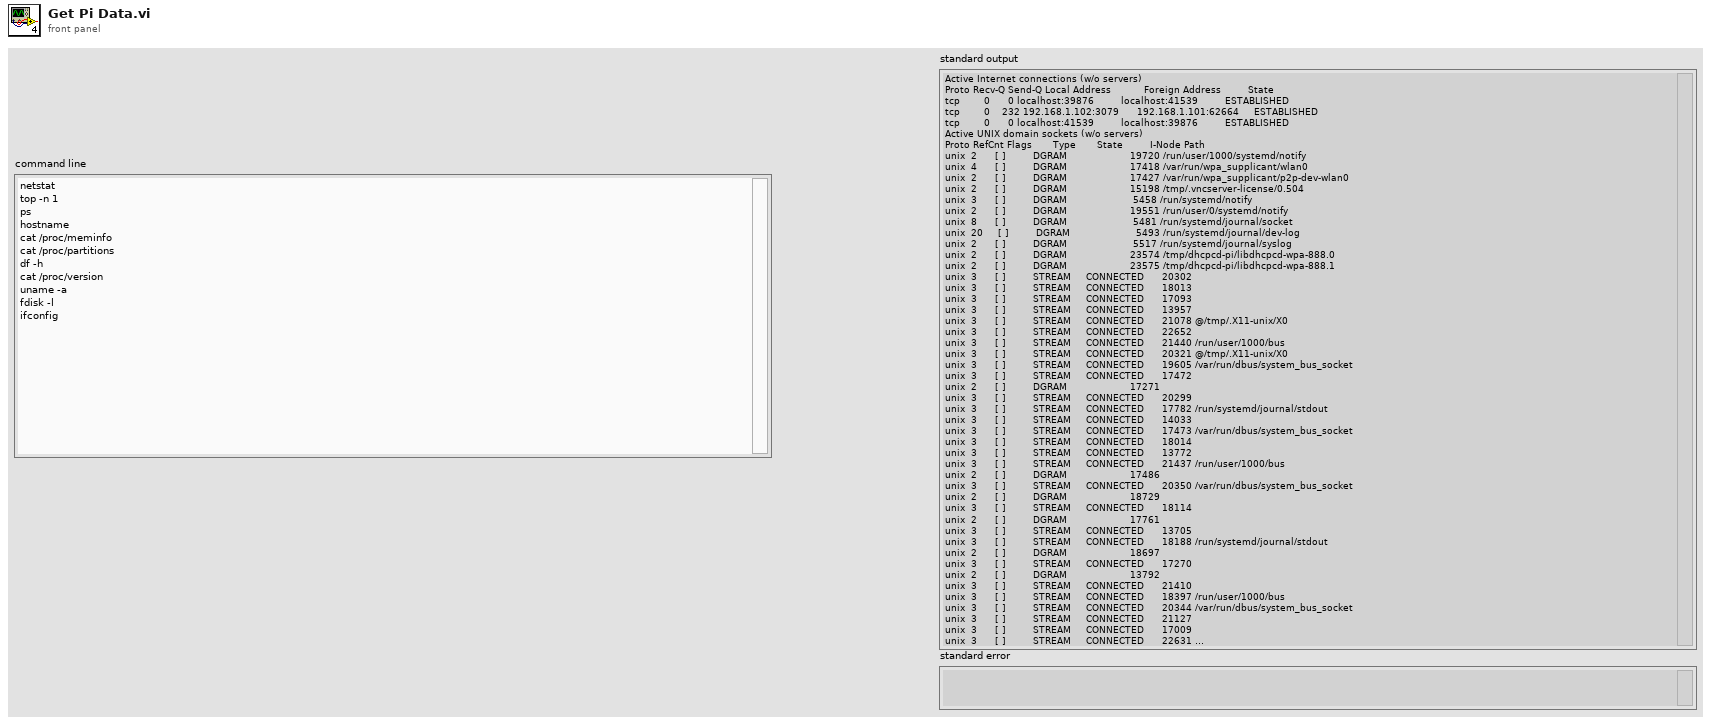
[diagram p1: front panel]
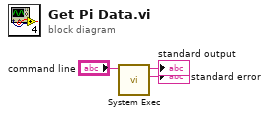
[diagram p0: block diagram]
diagram:
  n1 = call <vilib>:"System Exec.vi"("command line"="command line") -> ("standard error"=→"standard error":string, "standard output"=→"standard output":string)  [unwired: 7 in, 2 out]
